vi "20170509-lecture4-1 web.vi"() -> ()   [LabVIEW 2014]
panel:
  in  "URL":string
  in  "WebBrowser":refnum<k7>(container)
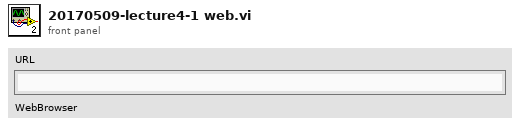
[diagram p1: front panel]
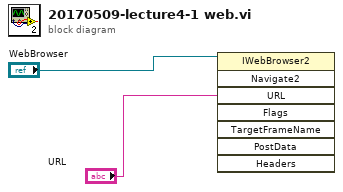
[diagram p0: block diagram]
diagram:
  n1 = invoke class="IWebBrowser2" method="Navigate2"(reference="WebBrowser", "URL"="URL") -> ()  [unwired: 6 in, 8 out]
